vi "Eval_SglVar_BulkMode.vi"(8 "error in (no error)":errorcluster, 9 "varValue":dbl[](array[numeric]) format="%#_13g", 11 "mupExpr in":refnum<data-value>) -> (0 "error out":errorcluster, 2 "Result":dbl[](array[numeric]), 3 "mupExpr out":refnum<data-value>)   [LabVIEW 2015, in "mupExpr.lvclass"]
doc: "Updates the value of the selected single variable then evaluates the expression in bulk mode. Returns the array of results.\n\nIf the expression contains no variables, the input values are ignored.\n\nIf the expression contains more than one variable only the \"Single Variable\" is updated.\n\nIf multiple expressions have been input, the last one in the list is evaluated."
uses:
  mupExpr.lvclass
  mupExpr.lvclass/mupExpr.ctl
  mupLib/mupCheckError.vi
  mupLib/mupLibPath.vi
  <vilib>/Utility/error.llb/Error Cluster From Error Code.vi
  mupLib/mupLib.lvlib
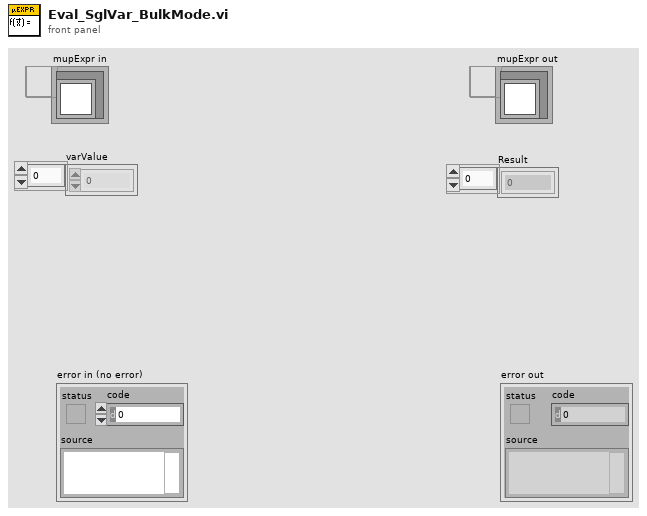
[diagram p1: front panel]
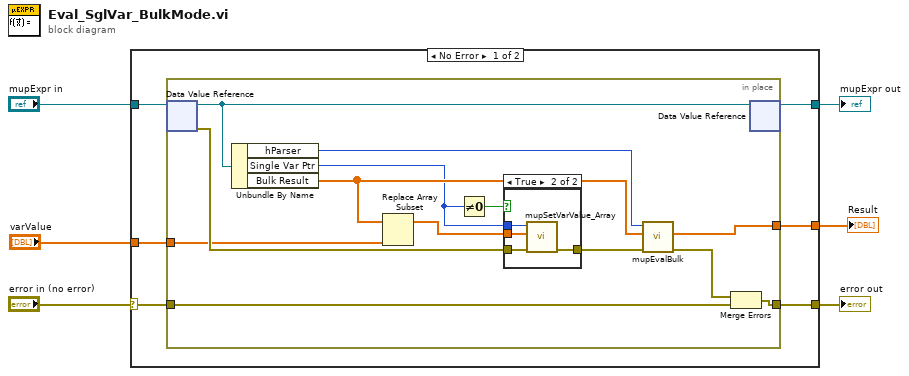
[diagram p0: block diagram]
diagram:
  n1 = case shown="No Error" "error in (no error)" {
    selector: "error in (no error)" -> [w12 w32]
    tunnel: [w10 w32] -> w5
    tunnel: [w7 w31] -> w3
    tunnel: "mupExpr in" -> [w8 w31]
    tunnel: "varValue" -> [w11 _]
    tunnel: [w9 _] -> w1
    frame No Error {
      n2 = in-place {
        in-place-border: w12 -> [w21]
        in-place-border: w11 -> [w17]
        in-place-border: [w19] -> w10
        in-place-border: [w25] -> w9
        n3 = in-place-dvr #1(w8) -> (w22:refnum<class "mupExpr.lvclass">, w23:errorcluster)
        n4 = Unbundle By Name(w22) -> ("hParser"=w24:u64, "Single Var Ptr"=w14:u64, "Bulk Result"=w18:dbl[])
        n5 = Replace Array Subset(array=w18, new element=w17) -> (w15:dbl[])  [unwired: 1 in]
        n6 = Not Equal To 0?(x=w14) -> (x != 0?=w13:bool)
        n7 = case shown="True" w13 {
          tunnel: w23 -> [w26 w30]
          tunnel: [w26 w29] -> w16
          tunnel: w15 -> [_ w28]
          tunnel: w14 -> [_ w27]
          frame False {
          }
          frame True {
            n8 = call "mupSetVarValue_Array.vi"("error in (no error)"=w30, "varValue"=w28, "varPtr in"=w27) -> ("error out"=w29:errorcluster)  [unwired: 7 in, 1 out]
          }
        }
        n9 = call "mupEvalBulk.vi"("error in (no error)"=w16, "a_res"=w18, "hParser in"=w24) -> ("error out"=w20:errorcluster, "results"=w25:dbl[])  [unwired: 6 in, 1 out]
        n10 = Merge Errors(w20, w21) -> (w19:errorcluster)
        n11 = in-place-dvr #1(w22) -> (w7:refnum<data-value>)  [unwired: 1 out]
      }
    }
    frame Error {
    }
  }
  "error out" <- w5
  "mupExpr out" <- w3
  "Result" <- w1
